vi "basement tank 3.vi"() -> ()   [LabVIEW 2019]
uses:
  <vilib>/NI/Current Value Table/Type Defs/Single Tag.ctl
  <vilib>/NI/Current Value Table/Type Defs/Data Types.ctl
  <vilib>/NI/STM/TCP/Read Meta Data (TCP Ref).vi
  <vilib>/NI/STM/TCP/Get Connection Reference (TCP).vi
  <vilib>/NI/AMC/Read Termination Message.vi
  <vilib>/NI/AMC/Create Single Message.vi
  <vilib>/NI/AMC/Update Message Routing Info.vi
  <vilib>/NI/STM/TCP/Read Meta Data (TCP Clst).vi
  <vilib>/NI/AMC/Globals.vi
  <vilib>/NI/STM/TCP/Write Message (TCP).vi
  <vilib>/NI/AMC/Send Message.vi
  <vilib>/NI/AMC/AMC.lvlib
  <vilib>/NI/STM/NI STM.lvlib
  <vilib>/NI/Current Value Table/Current Value Table.lvlib
panel:
  in  "Auto Level Main Tank":dbl(knob)=250.0 min=250.0 max=950.0 step=1.0 scale=200.0..1000.0 scale format="%#.3g"
  in  "Enable DI Auto Top-up":bool
  out "Boolean 7":bool
  out "Boolean 5":bool
  out "Boolean 2":bool
  in  "CuOAddAmount":dbl caption="CuO grams to add" min=-1000.0 max=1000.0 step=1.0
  out "Grams CuO to Add":dbl format="%.1f"
  in  "Dose Extra Oxide":bool
  in  "Sulfuric Proc 3":dbl=2.0 caption="ml Acid Proc 2" min=0.0 max=5000.0 step=1.0
  in  "Trig Sulfuric Proc 3":bool caption="Trigger Dose"
  out "Flow":bool
  in  "LEV Proc 3":dbl=2.0 caption="ml Lev Proc 2" min=0.0 max=1000.0 step=1.0
  in  "Trig Level Proc 3":bool caption="Trigger Dose"
  in  "UCON Proc 3":dbl=2.0 caption="ml UCON Proc 2" min=0.0 max=1000.0 step=1.0
  in  "Trig UCON Proc 3":bool caption="Trigger Dose"
  in  "SPS Proc 3":dbl=2.0 caption="ml SPS Proc 2" min=0.0 max=1000.0 step=1.0
  in  "Trig SPS Proc 3":bool caption="Trigger Dose"
  out "To Plating Process 5 & 6":bool
  out "ThreewayLowerElbow":bool
  out "PipeToTank":bool
  out "Tnk3Tee 2":bool
  out "PipeToPump 2":bool
  in  "BasT3_L Last Hr":bool
  out "BTnk1 SG":dbl format="%.3f"
  in  "BasT3_P Last Hr":bool
  out "Boiler Water Facilities Valve":dbl(slide) scale=0.0..100.0
  out "Tempered Water Facilities Valve":dbl(slide) scale=0.0..100.0
  out "Chilled Water Facilities Valve":dbl(slide) scale=0.0..100.0
  in  "Supply Pressure (kPa)":dbl(knob)=50.0 min=50.0 max=200.0 step=5.0 scale=50.0..200.0
  in  "BasT3_Flow Last Hr":bool
  out "Total Flow (when operated with plating tanks)":dbl(knob) scale=0.0..150.0
  in  "Specific Gravity":dbl(knob)=1.0 min=1.0 max=1.25 step=0.0025 scale=1.0..1.25
  out "Boiler Injection":u8(slide) scale=0.0..100.0
  out "Flow to Oxide Sys":dbl(slide) scale=0.0..10.0 scale format="%.1f"
  out "OxideToFilter":bool
  out "Oxide Pump":bool
  out "Boolean 4":bool
  out "OxideDose Indicate":bool
  in  "Flow rate To Oxide":dbl(knob)=2.0 min=2.0 max=12.0 step=0.1 scale=2.0..12.0
  in  "Oxide Dosing Enable":bool
  out "Chilled Injection":u8(slide) scale=0.0..100.0
  out "Tempered Injection":u8(slide) scale=0.0..100.0
  in  "BasT3_T Last Hr":bool
  in  "Enable T-Control":bool
  in  "Temperature Setpoint":dbl(knob)=15.0 min=15.0 max=85.0 step=0.1 scale=15.0..85.0 scale format="%#.1g"
  out "Boiler Water Out":dbl(knob) scale=10.0..110.0
  out "Boiler Water In":dbl(knob) scale=10.0..110.0
  out "Tempered Water Out":dbl(knob) scale=10.0..35.0
  out "Tempered Water In":dbl(knob) scale=10.0..35.0
  out "Chilled Water Out":dbl(knob) scale=0.0..25.0
  out "Chilled Water In":dbl(knob) scale=0.0..25.0
  in  "Tab Control":enum32{"Main Pump", "Lift Pump"}(tab)
  out "Amps":dbl format="%#.2g"
  out "Volts":dbl format="%#.1f"
  out "VFD T":dbl format="%#.2g"
  out "RPM":dbl format="%#.2f"
  out "Fault Code":dbl format="%#.2g"
  out "Freq":dbl format="%#.2g"
  out "Fault Code Ox Pmp":dbl caption="Fault Code" format="%#.2g"
  out "VFD T Ox Pmp":dbl caption="VFD T" format="%#.2g"
  out "Amps Ox Pmp":dbl caption="Amps" format="%#.2g"
  out "Volts Ox Pmp":dbl caption="Volts" format="%#.1f"
  out "Boolean 6":bool
  out "Circulator":bool
  out "HeatExchanger":bool
  out "Main Pump":bool
  out "Supply Pressure (kPa)":dbl(knob) scale=0.0..250.0
  out "Total Added":dbl format="%.2g"
  out "DI Flow (L/min)":dbl(knob) scale=0.0..100.0
  in  "Liters DI to Add":dbl(knob) min=0.0 max=500.0 step=1.0 scale=0.0..500.0
  in  "Add DI Water":bool
  in  "Drain System to Tree":bool
  in  "Enable Main Pump":bool
  out "E Stop":bool
  out "Run Enabled?":bool
  out "Supply Temperature":dbl(slide) scale=0.0..100.0
  out "Tank":dbl(slide) scale=0.0..1000.0
  in  "Machine":bool
  in  "Basement 4":bool
  in  "Dryer":bool
  in  "Rinse 4":bool
  in  "Rinse 3":bool
  in  "Rinse 2":bool
  in  "Basement 3":bool
  in  "Basement 2":bool
  in  "Basement 1":bool
  in  "Plater 6":bool
  in  "Plater 5":bool
  in  "Plater 4":bool
  in  "Plater 3":bool
  in  "Plater 2":bool
  in  "Plater 1":bool
  in  "Predip":bool
  in  "Rinse 1":bool
  in  "Cleaner":bool
  in  "Etch":bool
  out "status":string
  out "Tnk1Tee":bool
  out "PipeToPump":bool
  # "Module Selection"
  # "@"
  # "SG"
  # "T349"
  # "L/min"
  # "Dosing"
  # "SPS"
  # "UCON"
  # "Leveler"
  # "Sulfuric Acid"
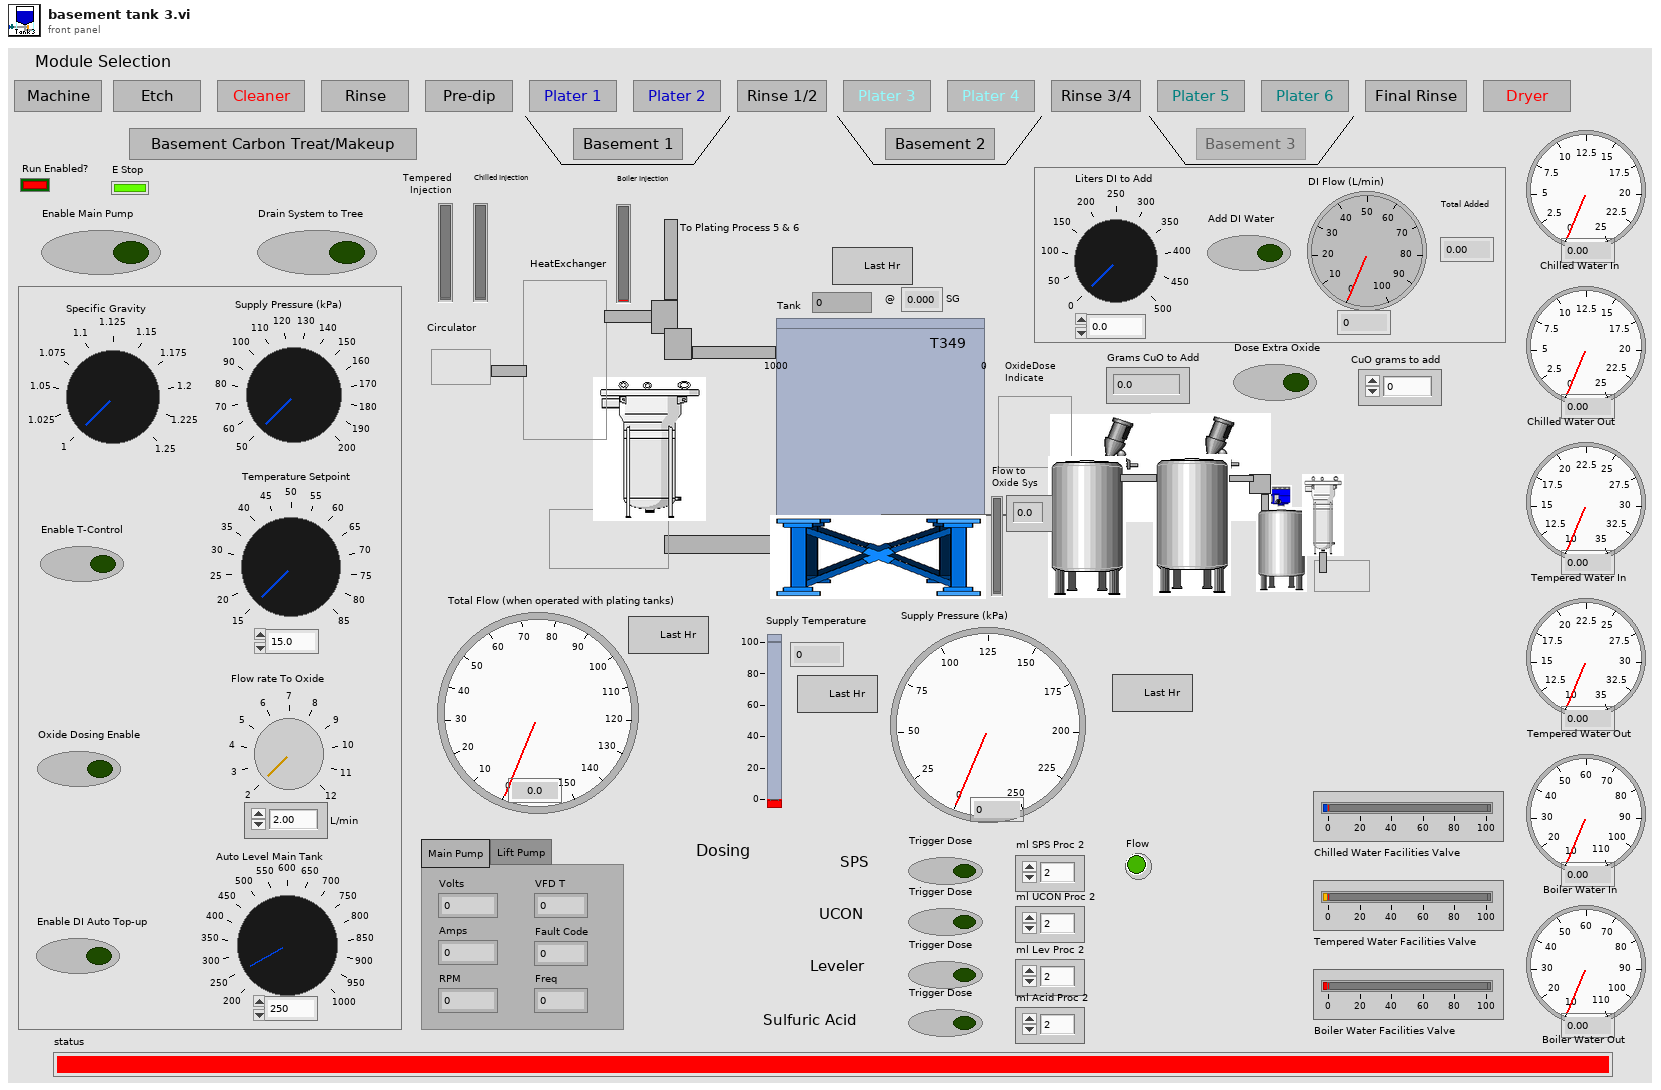
[diagram p1: front panel]
types:
  T1 = typedef "Current Value Table.lvlib/Single Tag.ctl" = cluster{"Data Type":T2, "Name":string, "Value":string, "Description":string}
  T2 = typedef "Current Value Table.lvlib/Data Types.ctl" = enum16{"Double", "Single", "I64", "I32", "I16", "I8", "U64", "U32", "U16", "U8", "String", "Boolean", "Array of U8", "Array of U16", "Array of U32", "Array of U64", "Array of I64", "Array of I32", "Array of I16", "Array of I8", "Array of Double", "Array of Single", "Array of Boolean", "Array of String"}
  T3 = typedef "NI STM.lvlib/TCP Connection Info.ctl" = cluster{"connection ID":refnum<k5>, "meta data":T4[]}
  T4 = typedef "NI STM.lvlib/MetaDataElement.ctl" = string
  T5 = typedef "AMC.lvlib/Message Queue.ctl" = refnum<queue>
  T6 = enum8{"Enabled", "Disabled", "Disabled and Grayed Out"}
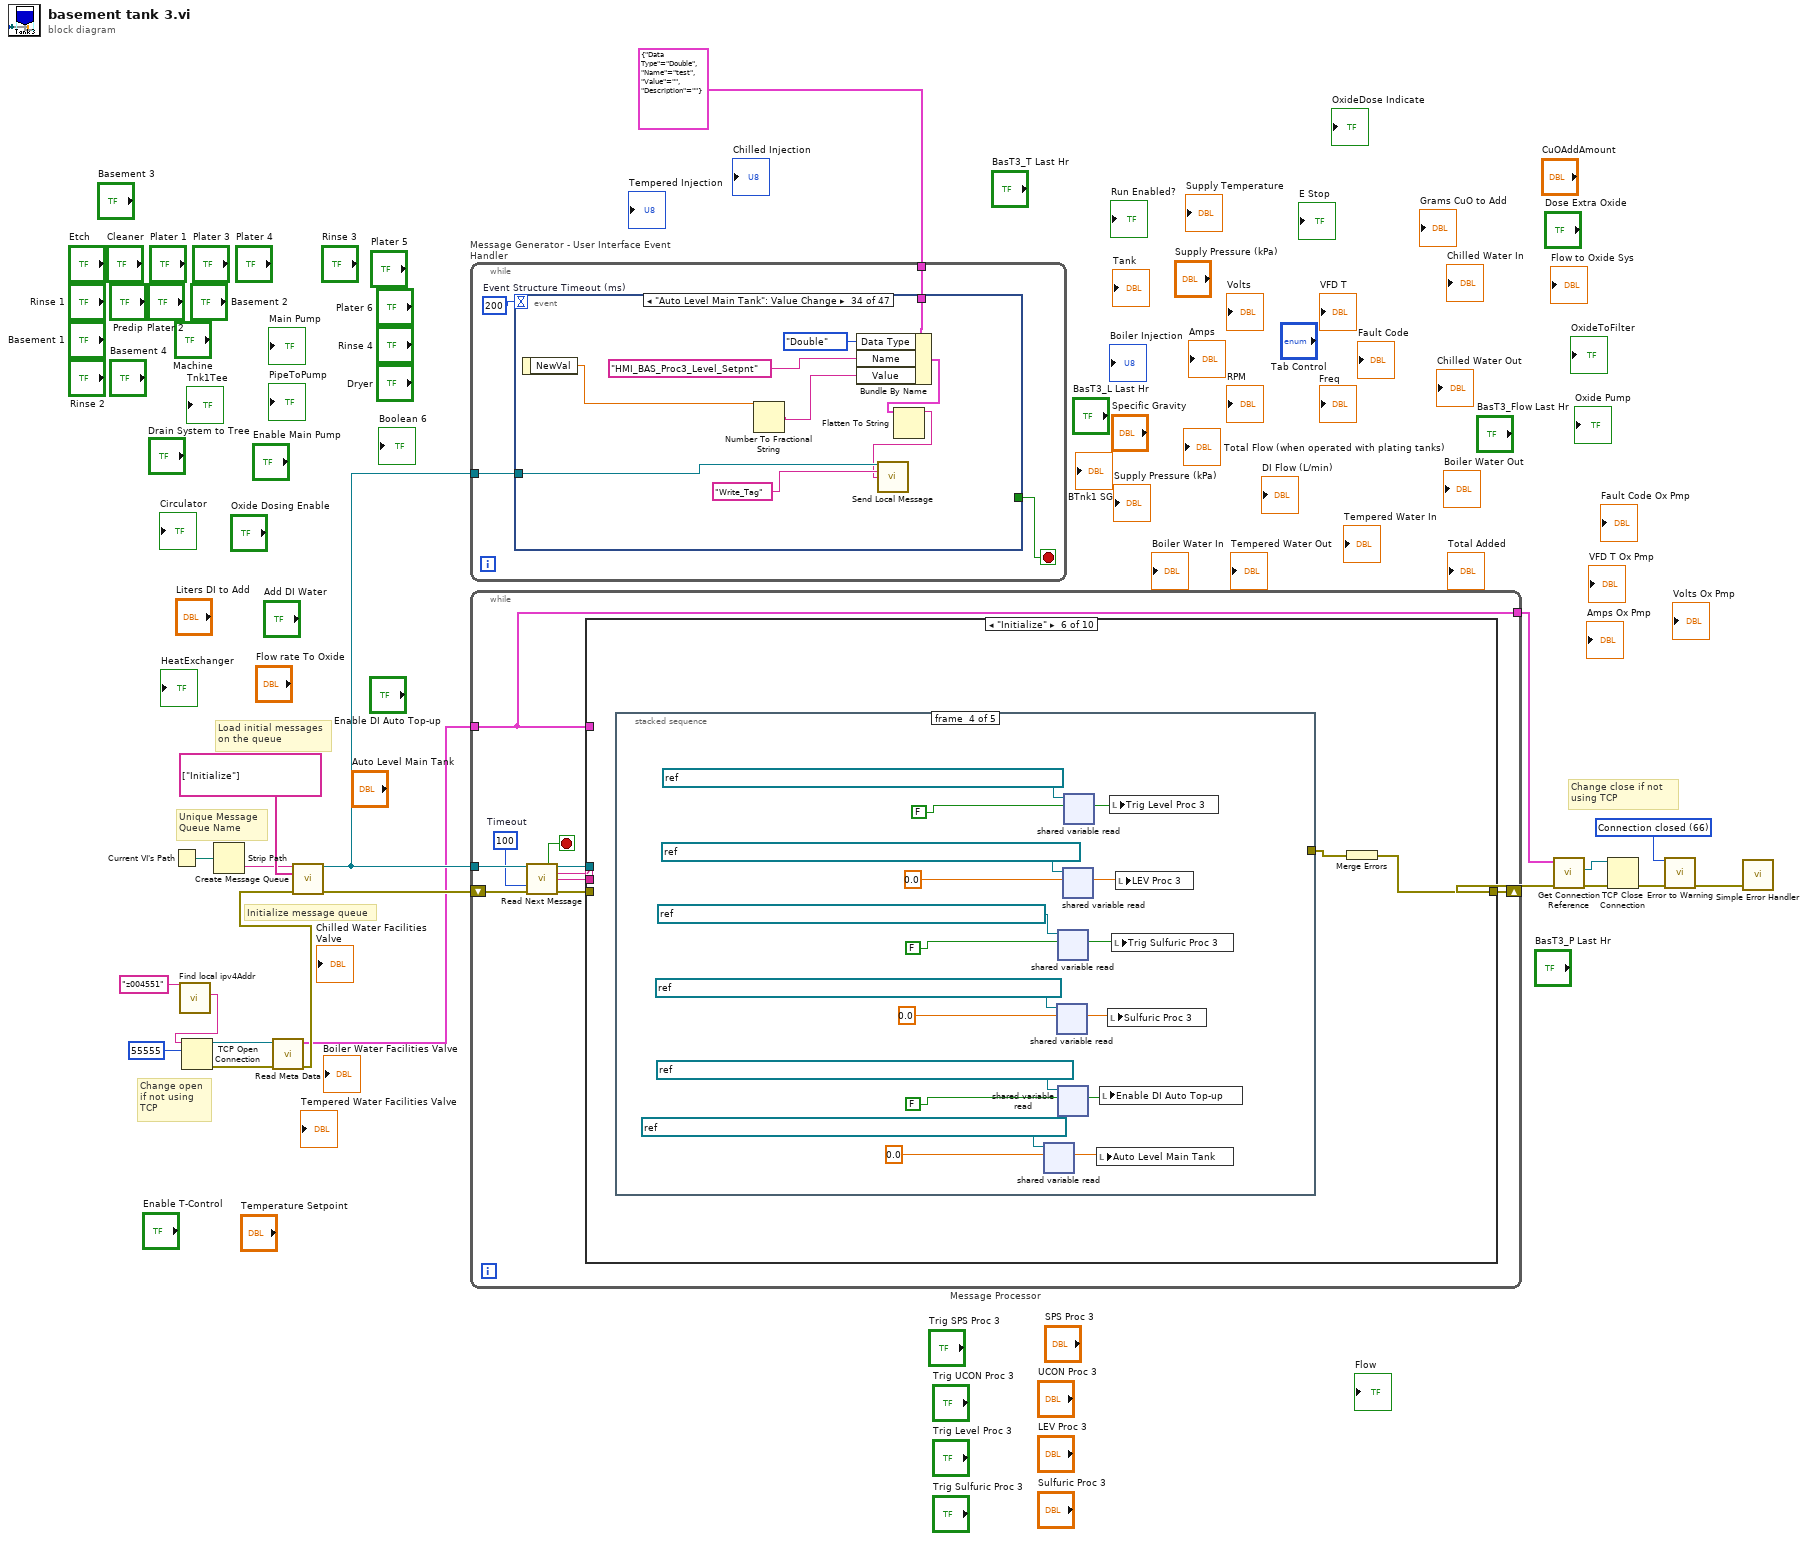
[diagram p0: block diagram]
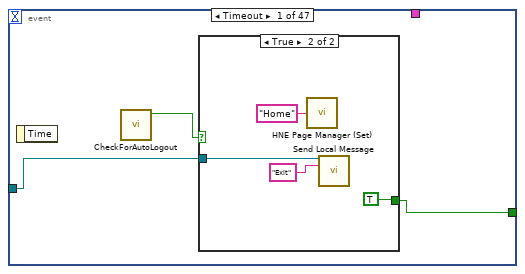
[diagram p2: hidden frame]
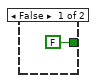
[diagram p3: hidden frame]
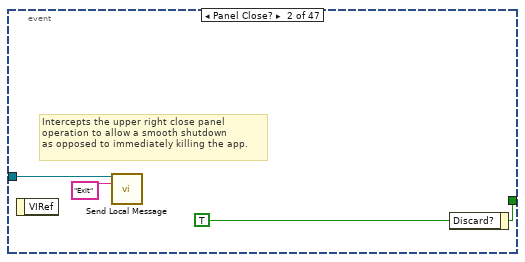
[diagram p4: hidden frame]
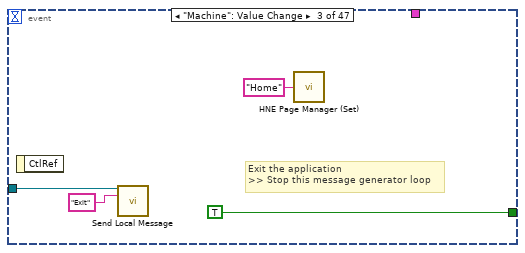
[diagram p5: hidden frame]
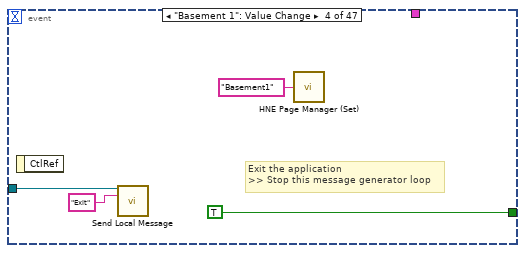
[diagram p6: hidden frame]
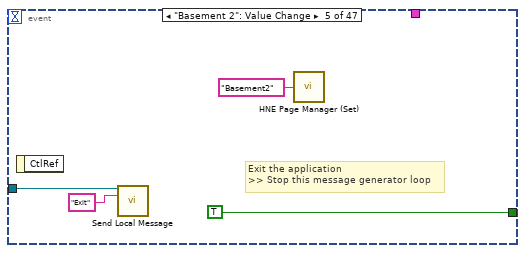
[diagram p7: hidden frame]
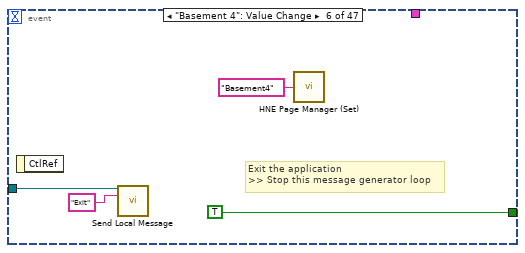
[diagram p8: hidden frame]
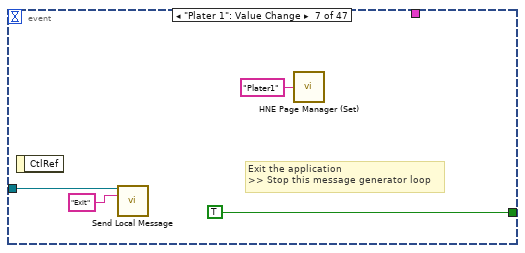
[diagram p9: hidden frame]
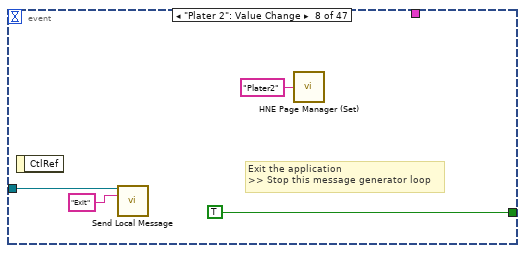
[diagram p10: hidden frame]
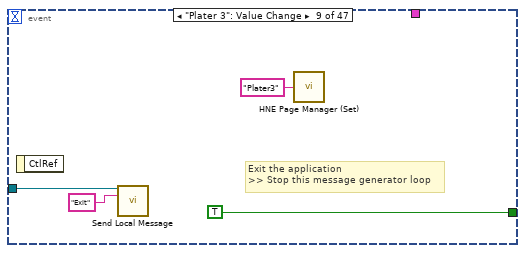
[diagram p11: hidden frame]
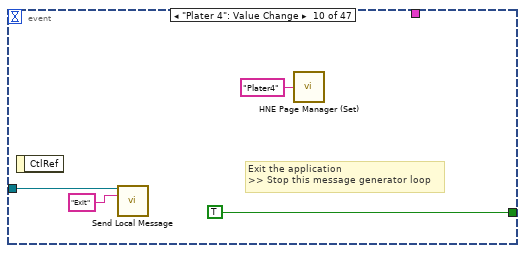
[diagram p12: hidden frame]
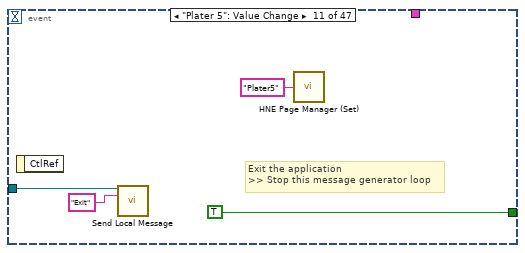
[diagram p13: hidden frame]
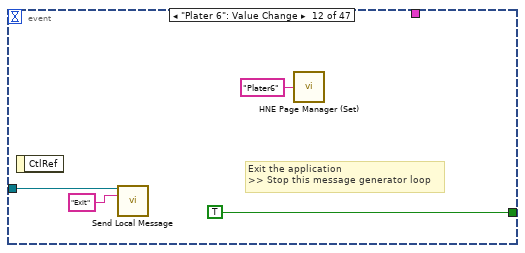
[diagram p14: hidden frame]
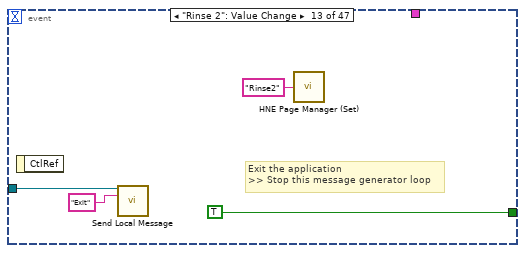
[diagram p15: hidden frame]
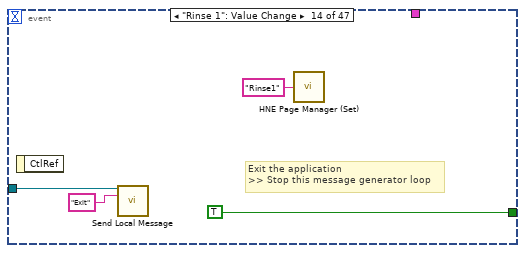
[diagram p16: hidden frame]
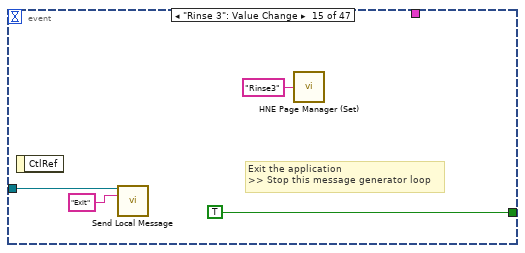
[diagram p17: hidden frame]
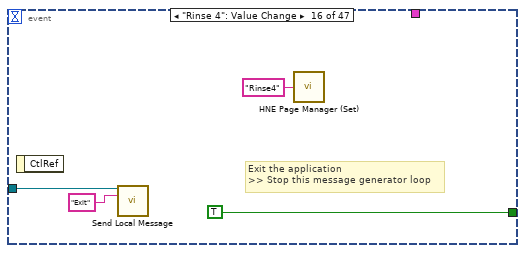
[diagram p18: hidden frame]
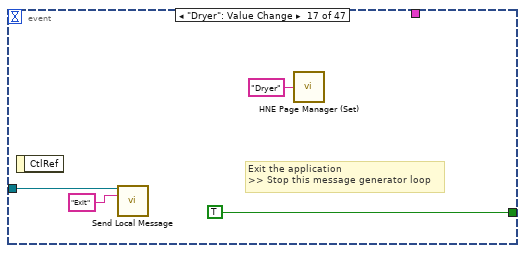
[diagram p19: hidden frame]
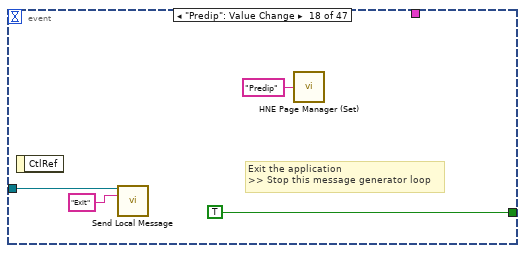
[diagram p20: hidden frame]
diagram:
  w9 = 66 items=["No Error", "Argument Error", "Memory Full", "Out of Zone", "End of File", "File Already Open", "Generic File IO Error", "File Not Found", "File Permission Error", "Disk Full", "Duplicate Path", "Too Many Files Open", "Not Enabled", "Resource File Not Found", "Cannot Add Resource", "Resource Not Found", "Image Not Found", "Image Memory Error", "Pen Does Not Exist", "Config Bad Type", "Config Token Not Found", "Config Parse Error", "Config Memory Error", "Bad External Code Format", "Bad External Code Offset", "External Code Not Present", "Null Window", "Destroy Window Mixup", "Null Menu", "Print Aborted", "Bad Print Record", "Print Driver Error", "Windows Error During Print", "Memory Error During Print", "Print Dialog Error", "Generic Print Error", "Invalid Device Refnum", "Device Not Found", "Device Parameter Error", "Device Unit Error", "Can't Open Device", "Device Call Aborted", "Generic Error", "Cancelled By User", "Object ID Too Low", "Object ID Too High", "Object Not In Heap", "Unknown Heap", "Bad DefProc ID", "DefProc Not In Table", "Message Out Of Range", "Null Method", "Unknown Message", "Manager Call Not Supported", "Bad address", "Connection In progress", "Connection timed out", "Connection is already in progress", "Network attribute not supported", "Network error", "Address in use", "System out of memory", "Connection aborted", "Connection refused", "Connection is not connected", "Connection is already connected", "Connection closed", "Initialize error (interapplication manager)", "Bad occurrence", "Wait on unbound occurrence handler", "Occurrence queue overflow", "Bad path", "Semaphore not signaled", "Unrecognized type (interapplication manager)"] ("1st Error to Convert")
  # "Change close if not using TCP"
  # "Change open if not using TCP"
  # "Initialize message queue"
  # "Unique Message\nQueue Name"
  # "Load initial messages\non the queue"
  n1 = Current VI's Path() -> (path=w16:path)
  n2 = call "Find local ipv4Addr.vi"("MachineToFind"="z004551" ("Target IP Address")) -> ("name"=w1:string)  [unwired: 9 in, 1 out]
  n3 = TCP Open Connection(address=w1, remote port or service name=u16 55555 ("remote port")) -> (connection ID=w14:refnum<k5>, error out=w13:errorcluster)  [unwired: 1 in, 2 out]
  n4 = Strip Path(path=w16) -> (name=w19:string)  [unwired: 1 out]
  n5 = call-poly <vilib>:"Read Meta Data.vi"("error in"=w13, "connection ID"=w14) -> ("error out"=w12:errorcluster, "connection info out"=w11:T3)  [unwired: 7 in, 1 out]
  n6 = call <vilib>:"Create Message Queue.vi"("message queue name"=w19, "initial message names"=string[] ["Initialize"], "error in"=w12) -> ("message queue out"=w18:T5, "error out"=w17:errorcluster)  [unwired: 11 in]
  n7 = while "Message Generator - User Interface Event Handler" {
    tunnel: w18 -> [w22]
    tunnel: T1 {"Data Type"=enum."Double", "Name"="test", "Value"="", "Description"=""} ("Tag") -> [w21]
    stop <- w23 stop-if-true
    w24 = 200  # Event Structure Timeout (ms)
    n8 = event shown="[33] \"Auto Level Main Tank\": Value Change" {
      selector: _ -> [_ _ _ _ _ _ _ _ _ _ _ _ _ _ _ _ _ _ _ _ _ _ _ _ _ _ _ _ _ _ _ _ _ _ _ _ _ _ _ _ _ _ _ _ _ _ _]
      dyn-events: _ -> [_ _ _ _ _ _ _ _ _ _ _ _ _ _ _ _ _ _ _ _ _ _ _ _ _ _ _ _ _ _ _ _ _ _ _ _ _ _ _ _ _ _ _ _ _ _ _]
      timeout: w24 -> [_ _ _ _ _ _ _ _ _ _ _ _ _ _ _ _ _ _ _ _ _ _ _ _ _ _ _ _ _ _ _ _ _ _ _ _ _ _ _ _ _ _ _ _ _ _ _]
      tunnel: [w25 w35 TRUE ("Discard?") TRUE ("Discard?") TRUE ("Discard?") TRUE ("Discard?") TRUE ("Discard?") TRUE ("Discard?") TRUE ("Discard?") TRUE ("Discard?") TRUE ("Discard?") TRUE ("Discard?") TRUE ("Discard?") TRUE ("Discard?") TRUE ("Discard?") TRUE ("Discard?") TRUE ("Discard?") TRUE ("Discard?") TRUE ("Discard?") TRUE ("Discard?") _ _ _ _ _ _ _ _ _ _ _ _ _ _ _ _ _ _ _ _ _ _ _ _ _ _ _] -> w23
      tunnel: w22 -> [w26 w33 w37 w41 w45 w49 w53 w57 w61 w65 w69 w73 w77 w81 w85 w89 w93 w97 w101 w105 w108 w119 w129 w139 w149 w159 w169 w179 w189 w199 w209 w219 w228 w237 w246 w255 w264 w273 w282 w291 w300 w309 w318 w319 w324 w329 w334]
      tunnel: w21 -> [_ _ _ _ _ _ _ _ _ _ _ _ _ _ _ _ _ _ _ _ _ w113 w123 w133 w143 w153 w163 w173 w183 w193 w203 w213 w224 w233 w242 w251 w260 w269 w278 w287 w296 w305 w314 _ _ _ _]
      event Timeout {
        n9 = event-data() -> ()  [unwired: 2 out]
        n10 = call "CheckForAutoLogout.vi"() -> ("Boolean"=w27:bool)  [unwired: 11 in]
        n11 = case shown="True" w27 {
          tunnel: [FALSE ("Discard?") TRUE ("Discard?")] -> w25
          tunnel: w26 -> [_ w29]
          frame False {
          }
          frame True {
            n12 = call <userlib>:"HNE Page Manager (Set).vi"("Next Page"="Home") -> ()  [unwired: 4 in, 1 out]
            n13 = call <vilib>:"Send Local Message.vi"("message queue in"=w29, "message name"="Exit") -> ()  [unwired: 11 in, 3 out]
          }
        }
      }
      event Panel Close? {
        w35 = TRUE ("Discard?")
        # "Intercepts the upper right close panel\noperation to allow a smooth shutdown\nas opposed to immediately killing the app."
        n14 = event-data() -> ()  [unwired: 2 out]
        n15 = call <vilib>:"Send Local Message.vi"("message queue in"=w33, "message name"="Exit") -> ()  [unwired: 11 in, 3 out]
        n16 = event-data("Discard?"=w35) -> ()  [unwired: 1 in, 1 out]
      }
      event "Machine": Value Change {
        # "Exit the application\n>> Stop this message generator loop"
        n17 = event-data() -> ()  [unwired: 2 out]
        n18 = call <vilib>:"Send Local Message.vi"("message queue in"=w37, "message name"="Exit") -> ()  [unwired: 11 in, 3 out]
        n19 = call <userlib>:"HNE Page Manager (Set).vi"("Next Page"="Home") -> ()  [unwired: 4 in, 1 out]
      }
      event "Basement 1": Value Change {
        # "Exit the application\n>> Stop this message generator loop"
        n20 = event-data() -> ()  [unwired: 2 out]
        n21 = call <vilib>:"Send Local Message.vi"("message queue in"=w41, "message name"="Exit") -> ()  [unwired: 11 in, 3 out]
        n22 = call <userlib>:"HNE Page Manager (Set).vi"("Next Page"="Basement1") -> ()  [unwired: 4 in, 1 out]
      }
      event "Basement 2": Value Change {
        # "Exit the application\n>> Stop this message generator loop"
        n23 = event-data() -> ()  [unwired: 2 out]
        n24 = call <vilib>:"Send Local Message.vi"("message queue in"=w45, "message name"="Exit") -> ()  [unwired: 11 in, 3 out]
        n25 = call <userlib>:"HNE Page Manager (Set).vi"("Next Page"="Basement2") -> ()  [unwired: 4 in, 1 out]
      }
      event "Basement 4": Value Change {
        # "Exit the application\n>> Stop this message generator loop"
        n26 = event-data() -> ()  [unwired: 2 out]
        n27 = call <vilib>:"Send Local Message.vi"("message queue in"=w49, "message name"="Exit") -> ()  [unwired: 11 in, 3 out]
        n28 = call <userlib>:"HNE Page Manager (Set).vi"("Next Page"="Basement4") -> ()  [unwired: 4 in, 1 out]
      }
      event "Plater 1": Value Change {
        # "Exit the application\n>> Stop this message generator loop"
        n29 = event-data() -> ()  [unwired: 2 out]
        n30 = call <vilib>:"Send Local Message.vi"("message queue in"=w53, "message name"="Exit") -> ()  [unwired: 11 in, 3 out]
        n31 = call <userlib>:"HNE Page Manager (Set).vi"("Next Page"="Plater1") -> ()  [unwired: 4 in, 1 out]
      }
      event "Plater 2": Value Change {
        # "Exit the application\n>> Stop this message generator loop"
        n32 = event-data() -> ()  [unwired: 2 out]
        n33 = call <vilib>:"Send Local Message.vi"("message queue in"=w57, "message name"="Exit") -> ()  [unwired: 11 in, 3 out]
        n34 = call <userlib>:"HNE Page Manager (Set).vi"("Next Page"="Plater2") -> ()  [unwired: 4 in, 1 out]
      }
      event "Plater 3": Value Change {
        # "Exit the application\n>> Stop this message generator loop"
        n35 = event-data() -> ()  [unwired: 2 out]
        n36 = call <vilib>:"Send Local Message.vi"("message queue in"=w61, "message name"="Exit") -> ()  [unwired: 11 in, 3 out]
        n37 = call <userlib>:"HNE Page Manager (Set).vi"("Next Page"="Plater3") -> ()  [unwired: 4 in, 1 out]
      }
      event "Plater 4": Value Change {
        # "Exit the application\n>> Stop this message generator loop"
        n38 = event-data() -> ()  [unwired: 2 out]
        n39 = call <vilib>:"Send Local Message.vi"("message queue in"=w65, "message name"="Exit") -> ()  [unwired: 11 in, 3 out]
        n40 = call <userlib>:"HNE Page Manager (Set).vi"("Next Page"="Plater4") -> ()  [unwired: 4 in, 1 out]
      }
      event "Plater 5": Value Change {
        # "Exit the application\n>> Stop this message generator loop"
        n41 = event-data() -> ()  [unwired: 2 out]
        n42 = call <vilib>:"Send Local Message.vi"("message queue in"=w69, "message name"="Exit") -> ()  [unwired: 11 in, 3 out]
        n43 = call <userlib>:"HNE Page Manager (Set).vi"("Next Page"="Plater5") -> ()  [unwired: 4 in, 1 out]
      }
      event "Plater 6": Value Change {
        # "Exit the application\n>> Stop this message generator loop"
        n44 = event-data() -> ()  [unwired: 2 out]
        n45 = call <vilib>:"Send Local Message.vi"("message queue in"=w73, "message name"="Exit") -> ()  [unwired: 11 in, 3 out]
        n46 = call <userlib>:"HNE Page Manager (Set).vi"("Next Page"="Plater6") -> ()  [unwired: 4 in, 1 out]
      }
      event "Rinse 2": Value Change {
        # "Exit the application\n>> Stop this message generator loop"
        n47 = event-data() -> ()  [unwired: 2 out]
        n48 = call <vilib>:"Send Local Message.vi"("message queue in"=w77, "message name"="Exit") -> ()  [unwired: 11 in, 3 out]
        n49 = call <userlib>:"HNE Page Manager (Set).vi"("Next Page"="Rinse2") -> ()  [unwired: 4 in, 1 out]
      }
      event "Rinse 1": Value Change {
        # "Exit the application\n>> Stop this message generator loop"
        n50 = event-data() -> ()  [unwired: 2 out]
        n51 = call <vilib>:"Send Local Message.vi"("message queue in"=w81, "message name"="Exit") -> ()  [unwired: 11 in, 3 out]
        n52 = call <userlib>:"HNE Page Manager (Set).vi"("Next Page"="Rinse1") -> ()  [unwired: 4 in, 1 out]
      }
      event "Rinse 3": Value Change {
        # "Exit the application\n>> Stop this message generator loop"
        n53 = event-data() -> ()  [unwired: 2 out]
        n54 = call <vilib>:"Send Local Message.vi"("message queue in"=w85, "message name"="Exit") -> ()  [unwired: 11 in, 3 out]
        n55 = call <userlib>:"HNE Page Manager (Set).vi"("Next Page"="Rinse3") -> ()  [unwired: 4 in, 1 out]
      }
      event "Rinse 4": Value Change {
        # "Exit the application\n>> Stop this message generator loop"
        n56 = event-data() -> ()  [unwired: 2 out]
        n57 = call <vilib>:"Send Local Message.vi"("message queue in"=w89, "message name"="Exit") -> ()  [unwired: 11 in, 3 out]
        n58 = call <userlib>:"HNE Page Manager (Set).vi"("Next Page"="Rinse4") -> ()  [unwired: 4 in, 1 out]
      }
      event "Dryer": Value Change {
        # "Exit the application\n>> Stop this message generator loop"
        n59 = event-data() -> ()  [unwired: 2 out]
        n60 = call <vilib>:"Send Local Message.vi"("message queue in"=w93, "message name"="Exit") -> ()  [unwired: 11 in, 3 out]
        n61 = call <userlib>:"HNE Page Manager (Set).vi"("Next Page"="Dryer") -> ()  [unwired: 4 in, 1 out]
      }
      event "Predip": Value Change {
        # "Exit the application\n>> Stop this message generator loop"
        n62 = event-data() -> ()  [unwired: 2 out]
        n63 = call <vilib>:"Send Local Message.vi"("message queue in"=w97, "message name"="Exit") -> ()  [unwired: 11 in, 3 out]
        n64 = call <userlib>:"HNE Page Manager (Set).vi"("Next Page"="Predip") -> ()  [unwired: 4 in, 1 out]
      }
      event "Cleaner": Value Change {
        # "Exit the application\n>> Stop this message generator loop"
        n65 = event-data() -> ()  [unwired: 2 out]
        n66 = call <vilib>:"Send Local Message.vi"("message queue in"=w101, "message name"="Exit") -> ()  [unwired: 11 in, 3 out]
        n67 = call <userlib>:"HNE Page Manager (Set).vi"("Next Page"="Clean") -> ()  [unwired: 4 in, 1 out]
      }
      event "Etch": Value Change {
        # "Exit the application\n>> Stop this message generator loop"
        n68 = event-data() -> ()  [unwired: 2 out]
        n69 = call <vilib>:"Send Local Message.vi"("message queue in"=w105, "message name"="Exit") -> ()  [unwired: 11 in, 3 out]
        n70 = call <userlib>:"HNE Page Manager (Set).vi"("Next Page"="Etch") -> ()  [unwired: 4 in, 1 out]
      }
      event Menu Selection (User) {
        # "Add run-time menu items to the message\nqueue. The message handler case names must match the menu ItemTag names."
        n71 = event-data() -> ("ItemTag"=w109:string)  [unwired: 1 out]
        n72 = call <vilib>:"Send Local Message.vi"("message queue in"=w108, "message name"=w109) -> ()  [unwired: 11 in, 3 out]
      }
      event "Enable Main Pump": Value Change {
        n73 = event-data() -> ("NewVal"=w112:bool)  [unwired: 1 out]
        n74 = Boolean To (0,1)(Boolean=w112) -> (0, 1=w118:i16)
        n75 = Number To Decimal String(number=w118) -> (decimal integer string=w117:string)  [unwired: 1 in]
        n76 = Bundle By Name(cluster=w113, "Data Type"=Data_Types."Boolean", "Name"="HMI_Enable_BTnk3_Pump", "Value"=w117) -> (w116:T1)
        n77 = Flatten To String(anything=w116) -> (data string=w110:string)  [unwired: 3 in, 2 out]
        n78 = call <vilib>:"Send Local Message.vi"("message queue in"=w119, "message name"="Write_Tag", "message value"=w110) -> ()  [unwired: 10 in, 3 out]
      }
      event "Drain System to Tree": Value Change {
        n79 = event-data() -> ("NewVal"=w122:bool)  [unwired: 1 out]
        n80 = Boolean To (0,1)(Boolean=w122) -> (0, 1=w128:i16)
        n81 = Number To Decimal String(number=w128) -> (decimal integer string=w127:string)  [unwired: 1 in]
        n82 = Bundle By Name(cluster=w123, "Data Type"=Data_Types."Boolean", "Name"="HMI_Drain_BTank3", "Value"=w127) -> (w126:T1)
        n83 = Flatten To String(anything=w126) -> (data string=w120:string)  [unwired: 3 in, 2 out]
        n84 = call <vilib>:"Send Local Message.vi"("message queue in"=w129, "message name"="Write_Tag", "message value"=w120) -> ()  [unwired: 10 in, 3 out]
      }
      event "Enable T-Control": Value Change {
        n85 = event-data() -> ("NewVal"=w132:bool)  [unwired: 1 out]
        n86 = Boolean To (0,1)(Boolean=w132) -> (0, 1=w138:i16)
        n87 = Number To Decimal String(number=w138) -> (decimal integer string=w137:string)  [unwired: 1 in]
        n88 = Bundle By Name(cluster=w133, "Data Type"=Data_Types."Boolean", "Name"="HMI_BAS_Tank3_TControl_Enable", "Value"=w137) -> (w136:T1)
        n89 = Flatten To String(anything=w136) -> (data string=w130:string)  [unwired: 3 in, 2 out]
        n90 = call <vilib>:"Send Local Message.vi"("message queue in"=w139, "message name"="Write_Tag", "message value"=w130) -> ()  [unwired: 10 in, 3 out]
      }
      event "Oxide Dosing Enable": Value Change {
        n91 = event-data() -> ("NewVal"=w142:bool)  [unwired: 1 out]
        n92 = Boolean To (0,1)(Boolean=w142) -> (0, 1=w148:i16)
        n93 = Number To Decimal String(number=w148) -> (decimal integer string=w147:string)  [unwired: 1 in]
        n94 = Bundle By Name(cluster=w143, "Data Type"=Data_Types."Boolean", "Name"="HMI_Proc3_Run_OxideSys", "Value"=w147) -> (w146:T1)
        n95 = Flatten To String(anything=w146) -> (data string=w140:string)  [unwired: 3 in, 2 out]
        n96 = call <vilib>:"Send Local Message.vi"("message queue in"=w149, "message name"="Write_Tag", "message value"=w140) -> ()  [unwired: 10 in, 3 out]
      }
      event "Trig SPS Proc 3": Value Change {
        n97 = event-data() -> ("NewVal"=w152:bool)  [unwired: 1 out]
        n98 = Boolean To (0,1)(Boolean=w152) -> (0, 1=w158:i16)
        n99 = Number To Decimal String(number=w158) -> (decimal integer string=w157:string)  [unwired: 1 in]
        n100 = Bundle By Name(cluster=w153, "Data Type"=Data_Types."Boolean", "Name"="HMI_Dose_SPS_Proc3", "Value"=w157) -> (w156:T1)
        n101 = Flatten To String(anything=w156) -> (data string=w150:string)  [unwired: 3 in, 2 out]
        n102 = call <vilib>:"Send Local Message.vi"("message queue in"=w159, "message name"="Write_Tag", "message value"=w150) -> ()  [unwired: 10 in, 3 out]
      }
      event "Trig UCON Proc 3": Value Change {
        n103 = event-data() -> ("NewVal"=w162:bool)  [unwired: 1 out]
        n104 = Boolean To (0,1)(Boolean=w162) -> (0, 1=w168:i16)
        n105 = Number To Decimal String(number=w168) -> (decimal integer string=w167:string)  [unwired: 1 in]
        n106 = Bundle By Name(cluster=w163, "Data Type"=Data_Types."Boolean", "Name"="HMI_Dose_UCON_Proc3", "Value"=w167) -> (w166:T1)
        n107 = Flatten To String(anything=w166) -> (data string=w160:string)  [unwired: 3 in, 2 out]
        n108 = call <vilib>:"Send Local Message.vi"("message queue in"=w169, "message name"="Write_Tag", "message value"=w160) -> ()  [unwired: 10 in, 3 out]
      }
      event "Trig Level Proc 3": Value Change {
        n109 = event-data() -> ("NewVal"=w172:bool)  [unwired: 1 out]
        n110 = Boolean To (0,1)(Boolean=w172) -> (0, 1=w178:i16)
        n111 = Number To Decimal String(number=w178) -> (decimal integer string=w177:string)  [unwired: 1 in]
        n112 = Bundle By Name(cluster=w173, "Data Type"=Data_Types."Boolean", "Name"="HMI_Dose_Leveler_Proc3", "Value"=w177) -> (w176:T1)
        n113 = Flatten To String(anything=w176) -> (data string=w170:string)  [unwired: 3 in, 2 out]
        n114 = call <vilib>:"Send Local Message.vi"("message queue in"=w179, "message name"="Write_Tag", "message value"=w170) -> ()  [unwired: 10 in, 3 out]
      }
      event "Trig Sulfuric Proc 3": Value Change {
        n115 = event-data() -> ("NewVal"=w182:bool)  [unwired: 1 out]
        n116 = Boolean To (0,1)(Boolean=w182) -> (0, 1=w188:i16)
        n117 = Number To Decimal String(number=w188) -> (decimal integer string=w187:string)  [unwired: 1 in]
        n118 = Bundle By Name(cluster=w183, "Data Type"=Data_Types."Boolean", "Name"="HMI_Dose_Acid_Proc3", "Value"=w187) -> (w186:T1)
        n119 = Flatten To String(anything=w186) -> (data string=w180:string)  [unwired: 3 in, 2 out]
        n120 = call <vilib>:"Send Local Message.vi"("message queue in"=w189, "message name"="Write_Tag", "message value"=w180) -> ()  [unwired: 10 in, 3 out]
      }
      event "Dose Extra Oxide": Value Change {
        n121 = event-data() -> ("NewVal"=w192:bool)  [unwired: 1 out]
        n122 = Boolean To (0,1)(Boolean=w192) -> (0, 1=w198:i16)
        n123 = Number To Decimal String(number=w198) -> (decimal integer string=w197:string)  [unwired: 1 in]
        n124 = Bundle By Name(cluster=w193, "Data Type"=Data_Types."Boolean", "Name"="HMI_Proc3_Add_CuOxide", "Value"=w197) -> (w196:T1)
        n125 = Flatten To String(anything=w196) -> (data string=w190:string)  [unwired: 3 in, 2 out]
        n126 = call <vilib>:"Send Local Message.vi"("message queue in"=w199, "message name"="Write_Tag", "message value"=w190) -> ()  [unwired: 10 in, 3 out]
      }
      event "Add DI Water": Value Change {
        n127 = event-data() -> ("NewVal"=w202:bool)  [unwired: 1 out]
        n128 = Boolean To (0,1)(Boolean=w202) -> (0, 1=w208:i16)
        n129 = Number To Decimal String(number=w208) -> (decimal integer string=w207:string)  [unwired: 1 in]
        n130 = Bundle By Name(cluster=w203, "Data Type"=Data_Types."Boolean", "Name"="HMI_BAS_Proc3_AddDIVolume", "Value"=w207) -> (w206:T1)
        n131 = Flatten To String(anything=w206) -> (data string=w200:string)  [unwired: 3 in, 2 out]
        n132 = call <vilib>:"Send Local Message.vi"("message queue in"=w209, "message name"="Write_Tag", "message value"=w200) -> ()  [unwired: 10 in, 3 out]
      }
      event "Enable DI Auto Top-up": Value Change {
        n133 = event-data() -> ("NewVal"=w212:bool)  [unwired: 1 out]
        n134 = Boolean To (0,1)(Boolean=w212) -> (0, 1=w218:i16)
        n135 = Number To Decimal String(number=w218) -> (decimal integer string=w217:string)  [unwired: 1 in]
        n136 = Bundle By Name(cluster=w213, "Data Type"=Data_Types."Boolean", "Name"="HMI_BAS_Proc3_Level_Auto", "Value"=w217) -> (w216:T1)
        n137 = Flatten To String(anything=w216) -> (data string=w210:string)  [unwired: 3 in, 2 out]
        n138 = call <vilib>:"Send Local Message.vi"("message queue in"=w219, "message name"="Write_Tag", "message value"=w210) -> ()  [unwired: 10 in, 3 out]
      }
      event "Liters DI to Add": Value Change {
        n139 = event-data() -> ("NewVal"=w221:dbl)  [unwired: 1 out]
        n140 = Number To Fractional String(number=w221) -> (F-format string=w220:string)  [unwired: 3 in]
        n141 = Bundle By Name(cluster=w224, "Data Type"=Data_Types."Double", "Name"="HMI_BAS_Proc3_DI_Setpnt", "Value"=w220) -> (w227:T1)
        n142 = Flatten To String(anything=w227) -> (data string=w222:string)  [unwired: 3 in, 2 out]
        n143 = call <vilib>:"Send Local Message.vi"("message queue in"=w228, "message name"="Write_Tag", "message value"=w222) -> ()  [unwired: 10 in, 3 out]
      }
      event "Auto Level Main Tank": Value Change {
        n144 = event-data() -> ("NewVal"=w230:dbl)  [unwired: 1 out]
        n145 = Number To Fractional String(number=w230) -> (F-format string=w229:string)  [unwired: 3 in]
        n146 = Bundle By Name(cluster=w233, "Data Type"=Data_Types."Double", "Name"="HMI_BAS_Proc3_Level_Setpnt", "Value"=w229) -> (w236:T1)
        n147 = Flatten To String(anything=w236) -> (data string=w231:string)  [unwired: 3 in, 2 out]
        n148 = call <vilib>:"Send Local Message.vi"("message queue in"=w237, "message name"="Write_Tag", "message value"=w231) -> ()  [unwired: 10 in, 3 out]
      }
      event "Temperature Setpoint": Value Change {
        n149 = event-data() -> ("NewVal"=w239:dbl)  [unwired: 1 out]
        n150 = Number To Fractional String(number=w239) -> (F-format string=w238:string)  [unwired: 3 in]
        n151 = Bundle By Name(cluster=w242, "Data Type"=Data_Types."Double", "Name"="HMI_BAS_TNK3_T_Setpoint", "Value"=w238) -> (w245:T1)
        n152 = Flatten To String(anything=w245) -> (data string=w240:string)  [unwired: 3 in, 2 out]
        n153 = call <vilib>:"Send Local Message.vi"("message queue in"=w246, "message name"="Write_Tag", "message value"=w240) -> ()  [unwired: 10 in, 3 out]
      }
      event "Supply Pressure (kPa)": Value Change {
        n154 = event-data() -> ("NewVal"=w248:dbl)  [unwired: 1 out]
        n155 = Number To Fractional String(number=w248) -> (F-format string=w247:string)  [unwired: 3 in]
        n156 = Bundle By Name(cluster=w251, "Data Type"=Data_Types."Double", "Name"="HMI_BAS_TNK3_P_Setpoint", "Value"=w247) -> (w254:T1)
        n157 = Flatten To String(anything=w254) -> (data string=w249:string)  [unwired: 3 in, 2 out]
        n158 = call <vilib>:"Send Local Message.vi"("message queue in"=w255, "message name"="Write_Tag", "message value"=w249) -> ()  [unwired: 10 in, 3 out]
      }
      event "Flow rate To Oxide": Value Change {
        n159 = event-data() -> ("NewVal"=w257:dbl)  [unwired: 1 out]
        n160 = Number To Fractional String(number=w257) -> (F-format string=w256:string)  [unwired: 3 in]
        n161 = Bundle By Name(cluster=w260, "Data Type"=Data_Types."Double", "Name"="HMI_Proc3_OxFlow_SetPnt", "Value"=w256) -> (w263:T1)
        n162 = Flatten To String(anything=w263) -> (data string=w258:string)  [unwired: 3 in, 2 out]
        n163 = call <vilib>:"Send Local Message.vi"("message queue in"=w264, "message name"="Write_Tag", "message value"=w258) -> ()  [unwired: 10 in, 3 out]
      }
      event "Specific Gravity": Value Change {
        n164 = event-data() -> ("NewVal"=w266:dbl)  [unwired: 1 out]
        n165 = Number To Fractional String(number=w266) -> (F-format string=w265:string)  [unwired: 3 in]
        n166 = Bundle By Name(cluster=w269, "Data Type"=Data_Types."Double", "Name"="HMI_BAS_Proc3_Tank_SG", "Value"=w265) -> (w272:T1)
        n167 = Flatten To String(anything=w272) -> (data string=w267:string)  [unwired: 3 in, 2 out]
        n168 = call <vilib>:"Send Local Message.vi"("message queue in"=w273, "message name"="Write_Tag", "message value"=w267) -> ()  [unwired: 10 in, 3 out]
      }
      event "SPS Proc 3": Value Change {
        n169 = event-data() -> ("NewVal"=w275:dbl)  [unwired: 1 out]
        n170 = Number To Fractional String(number=w275) -> (F-format string=w274:string)  [unwired: 3 in]
        n171 = Bundle By Name(cluster=w278, "Data Type"=Data_Types."Double", "Name"="HMI_SPS_Amount_Proc3", "Value"=w274) -> (w281:T1)
        n172 = Flatten To String(anything=w281) -> (data string=w276:string)  [unwired: 3 in, 2 out]
        n173 = call <vilib>:"Send Local Message.vi"("message queue in"=w282, "message name"="Write_Tag", "message value"=w276) -> ()  [unwired: 10 in, 3 out]
      }
      event "UCON Proc 3": Value Change {
        n174 = event-data() -> ("NewVal"=w284:dbl)  [unwired: 1 out]
        n175 = Number To Fractional String(number=w284) -> (F-format string=w283:string)  [unwired: 3 in]
        n176 = Bundle By Name(cluster=w287, "Data Type"=Data_Types."Double", "Name"="HMI_UCON_Amount_Proc3", "Value"=w283) -> (w290:T1)
        n177 = Flatten To String(anything=w290) -> (data string=w285:string)  [unwired: 3 in, 2 out]
        n178 = call <vilib>:"Send Local Message.vi"("message queue in"=w291, "message name"="Write_Tag", "message value"=w285) -> ()  [unwired: 10 in, 3 out]
      }
      event "LEV Proc 3": Value Change {
        n179 = event-data() -> ("NewVal"=w293:dbl)  [unwired: 1 out]
        n180 = Number To Fractional String(number=w293) -> (F-format string=w292:string)  [unwired: 3 in]
        n181 = Bundle By Name(cluster=w296, "Data Type"=Data_Types."Double", "Name"="HMI_Leveler_Amount_Proc3", "Value"=w292) -> (w299:T1)
        n182 = Flatten To String(anything=w299) -> (data string=w294:string)  [unwired: 3 in, 2 out]
        n183 = call <vilib>:"Send Local Message.vi"("message queue in"=w300, "message name"="Write_Tag", "message value"=w294) -> ()  [unwired: 10 in, 3 out]
      }
      event "Sulfuric Proc 3": Value Change {
        n184 = event-data() -> ("NewVal"=w302:dbl)  [unwired: 1 out]
        n185 = Number To Fractional String(number=w302) -> (F-format string=w301:string)  [unwired: 3 in]
        n186 = Bundle By Name(cluster=w305, "Data Type"=Data_Types."Double", "Name"="HMI_Acid_Amount_Proc3", "Value"=w301) -> (w308:T1)
        n187 = Flatten To String(anything=w308) -> (data string=w303:string)  [unwired: 3 in, 2 out]
        n188 = call <vilib>:"Send Local Message.vi"("message queue in"=w309, "message name"="Write_Tag", "message value"=w303) -> ()  [unwired: 10 in, 3 out]
      }
      event "CuOAddAmount": Value Change {
        n189 = event-data() -> ("NewVal"=w311:dbl)  [unwired: 1 out]
        n190 = Number To Fractional String(number=w311) -> (F-format string=w310:string)  [unwired: 3 in]
        n191 = Bundle By Name(cluster=w314, "Data Type"=Data_Types."Double", "Name"="HMI_Proc3_CuOxideAddAmnt", "Value"=w310) -> (w317:T1)
        n192 = Flatten To String(anything=w317) -> (data string=w312:string)  [unwired: 3 in, 2 out]
        n193 = call <vilib>:"Send Local Message.vi"("message queue in"=w318, "message name"="Write_Tag", "message value"=w312) -> ()  [unwired: 10 in, 3 out]
      }
      event "BasT3_T Last Hr": Value Change {
        n194 = event-data() -> ("NewVal"=w320:bool)  [unwired: 6 out]
        n195 = case shown="True" w320 {
          tunnel: w319 -> [_ w323]
          frame False {
          }
          frame True {
            n196 = call <vilib>:"Send Local Message.vi"("message queue in"=w323, "message name"="DisplayLastHr", "message value"="BAS_Proc3_T") -> ()  [unwired: 10 in, 3 out]
          }
        }
      }
      event "BasT3_Flow Last Hr": Value Change {
        n197 = event-data() -> ("NewVal"=w325:bool)  [unwired: 6 out]
        n198 = case shown="True" w325 {
          tunnel: w324 -> [_ w328]
          frame False {
          }
          frame True {
            n199 = call <vilib>:"Send Local Message.vi"("message queue in"=w328, "message name"="DisplayLastHr", "message value"="BAS_Proc3_Total_Flow") -> ()  [unwired: 10 in, 3 out]
          }
        }
      }
      event "BasT3_P Last Hr": Value Change {
        n200 = event-data() -> ("NewVal"=w330:bool)  [unwired: 6 out]
        n201 = case shown="True" w330 {
          tunnel: w329 -> [_ w333]
          frame False {
          }
          frame True {
            n202 = call <vilib>:"Send Local Message.vi"("message queue in"=w333, "message name"="DisplayLastHr", "message value"="BAS_Proc3_P") -> ()  [unwired: 10 in, 3 out]
          }
        }
      }
      event "BasT3_L Last Hr": Value Change {
        n203 = event-data() -> ("NewVal"=w335:bool)  [unwired: 6 out]
        n204 = case shown="True" w335 {
          tunnel: w334 -> [_ w338]
          frame False {
          }
          frame True {
            n205 = call <vilib>:"Send Local Message.vi"("message queue in"=w338, "message name"="DisplayLastHr", "message value"="BAS_Proc3_Tank_Level") -> ()  [unwired: 10 in, 3 out]
          }
        }
      }
    }
  }
  n206 = while "Message Processor" {
    shift-left: w17 -> [w344]
    shift-right: [w348] -> w4
    tunnel: w18 -> [w345]
    tunnel: w11 -> [w339]
    tunnel: [w339] -> w5
    stop <- w347 stop-if-true
    w340 = 100  # Timeout
    n207 = call <vilib>:"Read Next Message.vi"("message queue in"=w345, "timeout (1 ms)"=w340, "error in"=w344) -> ("exit process?"=w347:bool, "message queue out"=w346:T5, "message name"=w342:string, "message value"=w341:string, "error out"=w343:errorcluster)  [unwired: 5 in, 3 out]
    n208 = case shown="\"Initialize\"" w342 {
      selector: w342 -> [_ _ w395 _ _ _ _ _ _ _]
      tunnel: w346 -> [_ _ _ _ _ _ w469 _ _ _]
      tunnel: w343 -> [w349 _ w396 w397 w399 _ w470 w472 w474 w478]
      tunnel: [w349 w351 w396 errorcluster {"status"=FALSE, "code"=0, "source"=""} ("error out") w399 w400 w468 w472 w473 w478] -> w348
      tunnel: w341 -> [_ _ _ _ _ _ _ _ w475 w479]
      tunnel: w339 -> [_ _ _ _ _ _ _ _ w477 _]
      frame "---------- Framework Operations ----------" {
        # "Dummy case to add a seperator in the Case Structure menu"
      }
      frame "", "Idle" {
        n209 = stacked-sequence {
          tunnel: [w359 _] -> w350
          frame #0 {
            n210 = shared-variable-read(refnum<k21> "ni.var.psp://z004551/CDL0100 ReadWriteTags/HMI_Drain_BTank3" ("shared variable refnum in"), FALSE) -> (w353:errorcluster, w356:bool)  [unwired: 1 in, 2 out]
            n211 = shared-variable-read(refnum<k21> "ni.var.psp://z004551/CDL0100 ReadWriteTags/HMI_BAS_Proc3_AddDIVolume" ("shared variable refnum in"), FALSE) -> (w360:errorcluster, w363:bool)  [unwired: 1 in, 2 out]
            n212 = shared-variable-read(refnum<k21> "ni.var.psp://z004551/CDL0100 ReadWriteTags/HMI_Enable_BTnk3_Pump" ("shared variable refnum in"), FALSE) -> (w361:errorcluster, w368:bool)  [unwired: 1 in, 2 out]
            n213 = call <userlib>:"Boolean Trigger__ogtk.vi"("Boolean Input"=w363) -> ("Falling Edge"=w362:bool)  [unwired: 1 in, 1 out]
            n214 = case shown="True" w356 {
              tunnel: [T6."Enabled" ("Disabled") T6."Disabled and Grayed Out" ("Disabled")] -> w355
              frame False {
              }
              frame True {
              }
            }
            n215 = case shown="True" w368 {
              tunnel: [T6."Enabled" ("Disabled") T6."Disabled and Grayed Out" ("Disabled")] -> w367
              frame False {
              }
              frame True {
              }
            }
            n216 = control-ref of="Drain System to Tree"() -> (w366:refnum<vi>)
            n217 = case shown="True" w362 {
              frame False {
              }
              frame True {
                n218 = local write "Add DI Water"(FALSE) -> ()
              }
            }
            n219 = control-ref of="Enable Main Pump"() -> (w354:refnum<vi>)
            n220 = property class="Bool (strict)"(reference=w366, "DisabledEnum"=w367) -> ()  [unwired: 1 in, 2 out]
            n221 = property class="Bool (strict)"(reference=w354, "DisabledEnum"=w355) -> ()  [unwired: 1 in, 2 out]
            n222 = Merge Errors(w361, w360, w353) -> (w359:errorcluster)
          }
          frame #1 {
            n223 = shared-variable-read(refnum<k21> "ni.var.psp://z004551/CDL0100 ReadTags/IO_Bas_Tnk3_3Way_At_Recirc" ("shared variable refnum in"), FALSE) -> (w384:bool)  [unwired: 1 in, 3 out]
            n224 = shared-variable-read(refnum<k21> "ni.var.psp://z004551/CDL0100 ReadTags/IO_Bas_Tnk3_3Way_At_Open" ("shared variable refnum in"), FALSE) -> (w386:bool)  [unwired: 1 in, 3 out]
            n225 = shared-variable-read(refnum<k21> "ni.var.psp://z004551/CDL0100 ReadTags/IO_Bas_Tnk3_3Way_At_Closed" ("shared variable refnum in"), FALSE) -> (w388:bool)  [unwired: 1 in, 3 out]
            n226 = shared-variable-read(refnum<k21> "ni.var.psp://z004551/CDL0100 ReadTags/BAS_Proc3_Oxide_FlowRate" ("shared variable refnum in"), 0.0) -> (w378:dbl)  [unwired: 1 in, 3 out]
            n227 = Or(x=w386, y=w384) -> (x .or. y?=→"ThreewayLowerElbow" →"PipeToTank":bool)
            n228 = Greater?(x=w378, y=1.0) -> (0:→"Boolean 4" →"Boolean 5" →"Boolean 2" →"Boolean 7":bool)
            n229 = Or(x=w388, y=w386) -> (x .or. y?=w383:bool)
            "To Plating Process 5 & 6" <- w383
            n230 = Or(x=w383, y=w384) -> (x .or. y?=→"PipeToPump 2" →"Tnk3Tee 2":bool)
          }
        }
        n231 = control-ref of="status"() -> (w352:refnum<vi>)
        n232 = call <userlib>:"TAE Format Alarm Ticker.vi"("Alarm Ticker Ref"=w352) -> ()  [unwired: 15 in]
        n233 = Merge Errors(w350) -> (w351:errorcluster)
      }
      frame "Missing Message Handler", Default {
        # "Call this case if a message is received that is not handled \nby any other case. Typically this is a programming error\nas a result of a typo or unhandled message/missing message handler."
        n234 = Format Into String(format string="DevError: Missing message handler for '%s\" message." ("message"), w395) -> (resulting string=w393:string)  [unwired: 2 in, 1 out]
        n235 = One Button Dialog(message=w393) -> ()  [unwired: 2 out]
      }
      frame "Error" {
        # "General Error Case - this case is called if an error is passed using the error cluster below. Typically most new errors should be handed in each individual case and not passed in the rror cluster. If necessary a custom error handler case should be added and called from other cases."
        n236 = call <vilib>:"Simple Error Handler.vi"("error in (no error)"=w397) -> ()  [unwired: 1 in, 8 out]
      }
      frame "---------- Generic Operations ----------" {
        # "Dummy case to add a seperator in the Case Structure menu"
      }
      frame "Initialize" {
        n237 = stacked-sequence {
          tunnel: [w411 _ _ _ _] -> w401
          frame #0 {
            n238 = shared-variable-read(refnum<k21> "ni.var.psp://z004551/CDL0100 ReadWriteTags/HMI_Drain_BTank3" ("shared variable refnum in"), FALSE) -> (w412:errorcluster, w414:bool)  [unwired: 1 in, 2 out]
            n239 = shared-variable-read(refnum<k21> "ni.var.psp://z004551/CDL0100 ReadWriteTags/HMI_BAS_Proc3_AddDIVolume" ("shared variable refnum in"), FALSE) -> (w405:bool)  [unwired: 1 in, 3 out]
            n240 = shared-variable-read(refnum<k21> "ni.var.psp://z004551/CDL0100 ReadWriteTags/HMI_Enable_BTnk3_Pump" ("shared variable refnum in"), FALSE) -> (w413:errorcluster, w417:bool)  [unwired: 1 in, 2 out]
            n241 = shared-variable-read(refnum<k21> "ni.var.psp://z004551/CDL0100 ReadWriteTags/HMI_BAS_Proc3_DI_Setpnt" ("shared variable refnum in"), 0.0) -> (w406:dbl)  [unwired: 1 in, 3 out]
            n242 = shared-variable-read(refnum<k21> "ni.var.psp://z004551/CDL0100 ReadWriteTags/HMI_BAS_Tank3_TControl_Enable" ("shared variable refnum in"), FALSE) -> (w402:bool)  [unwired: 1 in, 3 out]
            n243 = local write "Drain System to Tree"(w414) -> ()
            n244 = local write "Add DI Water"(w405) -> ()
            n245 = local write "Enable Main Pump"(w417) -> ()
            n246 = local write "Liters DI to Add"(w406) -> ()
            n247 = local write "Enable T-Control"(w402) -> ()
            n248 = Merge Errors(w413, w412) -> (w411:errorcluster)
          }
          frame #1 {
            n249 = shared-variable-read(refnum<k21> "ni.var.psp://z004551/CDL0100 ReadWriteTags/HMI_BAS_TNK3_P_Setpoint" ("shared variable refnum in"), 1.0) -> (w420:dbl)  [unwired: 1 in, 3 out]
            n250 = local write "Supply Pressure (kPa)"(w420) -> ()
          }
          frame #2 {
            n251 = shared-variable-read(refnum<k21> "ni.var.psp://z004551/CDL0100 ReadWriteTags/HMI_BAS_TNK3_T_Setpoint" ("shared variable refnum in"), 0.0) -> (w432:dbl)  [unwired: 1 in, 3 out]
            n252 = shared-variable-read(refnum<k21> "ni.var.psp://z004551/CDL0100 ReadWriteTags/HMI_BAS_Proc3_Tank_SG" ("shared variable refnum in"), 0.0) -> (w423:dbl)  [unwired: 1 in, 3 out]
            n253 = shared-variable-read(refnum<k21> "ni.var.psp://z004551/CDL0100 ReadWriteTags/HMI_Proc3_Run_OxideSys" ("shared variable refnum in"), FALSE) -> (w429:bool)  [unwired: 1 in, 3 out]
            n254 = shared-variable-read(refnum<k21> "ni.var.psp://z004551/CDL0100 ReadWriteTags/HMI_Proc3_OxFlow_SetPnt" ("shared variable refnum in"), 0.0) -> (w426:dbl)  [unwired: 1 in, 3 out]
            n255 = local write "Oxide Dosing Enable"(w429) -> ()
            n256 = local write "Temperature Setpoint"(w432) -> ()
            n257 = local write "Specific Gravity"(w423) -> ()
            n258 = local write "Flow rate To Oxide"(w426) -> ()
          }
          frame #3 {
            n259 = shared-variable-read(refnum<k21> "ni.var.psp://z004551/CDL0100 ReadWriteTags/HMI_BAS_Proc3_Level_Setpnt" ("shared variable refnum in"), 0.0) -> (w435:dbl)  [unwired: 1 in, 3 out]
            n260 = shared-variable-read(refnum<k21> "ni.var.psp://z004551/CDL0100 ReadWriteTags/HMI_Acid_Amount_Proc3" ("shared variable refnum in"), 0.0) -> (w442:dbl)  [unwired: 1 in, 3 out]
            n261 = shared-variable-read(refnum<k21> "ni.var.psp://z004551/CDL0100 ReadWriteTags/HMI_Dose_Acid_Proc3" ("shared variable refnum in"), FALSE) -> (w441:bool)  [unwired: 1 in, 3 out]
            n262 = shared-variable-read(refnum<k21> "ni.var.psp://z004551/CDL0100 ReadWriteTags/HMI_BAS_Proc3_Level_Auto" ("shared variable refnum in"), FALSE) -> (w438:bool)  [unwired: 1 in, 3 out]
            n263 = shared-variable-read(refnum<k21> "ni.var.psp://z004551/CDL0100 ReadWriteTags/HMI_Leveler_Amount_Proc3" ("shared variable refnum in"), 0.0) -> (w443:dbl)  [unwired: 1 in, 3 out]
            n264 = shared-variable-read(refnum<k21> "ni.var.psp://z004551/CDL0100 ReadWriteTags/HMI_Dose_Leveler_Proc3" ("shared variable refnum in"), FALSE) -> (w444:bool)  [unwired: 1 in, 3 out]
            n265 = local write "Auto Level Main Tank"(w435) -> ()
            n266 = local write "Enable DI Auto Top-up"(w438) -> ()
            n267 = local write "Sulfuric Proc 3"(w442) -> ()
            n268 = local write "Trig Level Proc 3"(w444) -> ()
            n269 = local write "Trig Sulfuric Proc 3"(w441) -> ()
            n270 = local write "LEV Proc 3"(w443) -> ()
          }
          frame #4 {
            n271 = shared-variable-read(refnum<k21> "ni.var.psp://z004551/CDL0100 ReadWriteTags/HMI_Dose_SPS_Proc3" ("shared variable refnum in"), FALSE) -> (w459:bool)  [unwired: 1 in, 3 out]
            n272 = shared-variable-read(refnum<k21> "ni.var.psp://z004551/CDL0100 ReadWriteTags/HMI_UCON_Amount_Proc3" ("shared variable refnum in"), 0.0) -> (w456:dbl)  [unwired: 1 in, 3 out]
            n273 = shared-variable-read(refnum<k21> "ni.var.psp://z004551/CDL0100 ReadWriteTags/HMI_Dose_UCON_Proc3" ("shared variable refnum in"), FALSE) -> (w457:bool)  [unwired: 1 in, 3 out]
            n274 = shared-variable-read(refnum<k21> "ni.var.psp://z004551/CDL0100 ReadWriteTags/HMI_Proc3_CuOxideAddAmnt" ("shared variable refnum in"), 0.0) -> (w453:dbl)  [unwired: 1 in, 3 out]
            n275 = shared-variable-read(refnum<k21> "ni.var.psp://z004551/CDL0100 ReadWriteTags/HMI_SPS_Amount_Proc3" ("shared variable refnum in"), 0.0) -> (w458:dbl)  [unwired: 1 in, 3 out]
            n276 = local write "Trig SPS Proc 3"(w459) -> ()
            n277 = local write "UCON Proc 3"(w456) -> ()
            n278 = local write "Trig UCON Proc 3"(w457) -> ()
            n279 = local write "CuOAddAmount"(w453) -> ()
            n280 = local write "SPS Proc 3"(w458) -> ()
          }
        }
        n281 = Merge Errors(w401) -> (w400:errorcluster)
      }
      frame "Exit" {
        # "Destroy message queue >> this will halt the UI event handler loop"
        # "Stop the VI\n>> Perform any cleanup tasks in this message case.\n>> Clear display before closing."
        n282 = call <vilib>:"Destroy Message Queue.vi"("message queue in"=w469, "error in"=w470) -> ("error out"=w468:errorcluster)  [unwired: 11 in, 2 out]
        n283 = local write "status"("" ("Status")) -> ()
      }
      frame "---------- Application Operations ----------" {
        # "Dummy case to add a seperator in the Case Structure menu"
      }
      frame "Write_Tag" {
        n284 = call-poly <vilib>:"Write Message.vi"("error in"=w474, "data"=w475, "name"="WriteTag", "connection info in"=w477) -> ("error out"=w473:errorcluster)  [unwired: 6 in, 1 out]
      }
      frame "DisplayLastHr" {
        n285 = call "Trace Variable 1 hour Popup.vi"("Tag"=w479) -> ()  [unwired: 11 in]
      }
    }
  }
  n286 = call-poly <vilib>:"Get Connection Reference.vi"("error in"=w4, "connection info in"=w5) -> ("error out"=w8:errorcluster, "connection ID out"=w7:refnum<k5>)  [unwired: 8 out]
  n287 = TCP Close Connection(connection ID=w7, error in (no error)=w8) -> (error out=w10:errorcluster)  [unwired: 2 out]
  n288 = call <vilib>:"Error to Warning.vi"("1st Error to Convert"=w9, "error in"=w10) -> ("warning out"=w6:errorcluster)  [unwired: 3 in, 10 out]
  n289 = call <vilib>:"Simple Error Handler.vi"("error in (no error)"=w6) -> ()  [unwired: 4 in, 5 out]
